vi "Analyze.vi"(8 "error in (no error)":errorcluster, 11 "HIJ Vision Display in":refnum<class "HIJ Vision Display.lvclass">) -> (0 "error out":errorcluster, 3 "HIJ Vision Display out":refnum<class "HIJ Vision Display.lvclass">)   [LabVIEW 2014, in "HIJ Vision Display.lvlib" / "HIJ Vision Display.lvclass"]
uses:
  HIJ Vision Display.lvclass
  <vilib>/vision/Image Controls.llb/IMAQ Image.ctl
  HIJ Vision Display.lvclass/HIJ Vision Display.ctl
  Analyze Actor/Analyze Actor Messages/Analyze Msg/Analyze Msg.lvclass/Analyze Msg.ctl
  <vilib>/ActorFramework/Message Enqueuer/Message Enqueuer.lvclass/Message Enqueuer.ctl
  <vilib>/ActorFramework/Message Enqueuer/Enqueue.vi
  <vilib>/ActorFramework/Message Priority Queue/Priority Enqueue.vi
  <vilib>/ActorFramework/Message Enqueuer/Message Enqueuer.lvclass
  Analyze Actor/Analyze Actor Messages/Analyze Msg/Analyze Msg.lvclass
panel:
  out "Image Out":T1
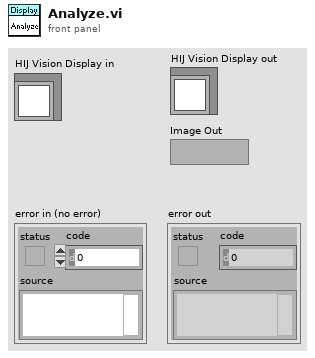
[diagram p1: front panel]
types:
  T1 = typedef "IMAQ Image.ctl" = refnum<image>
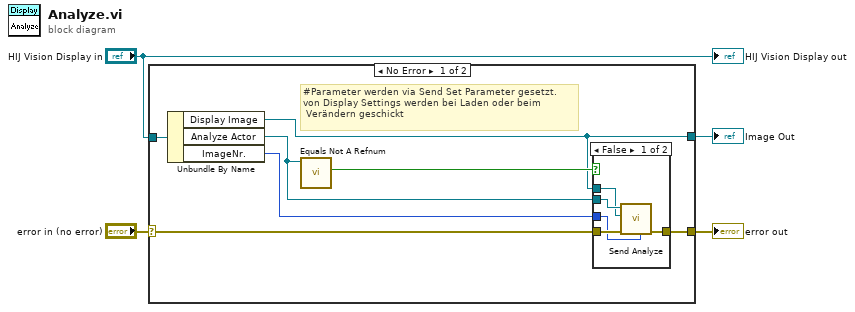
[diagram p0: block diagram]
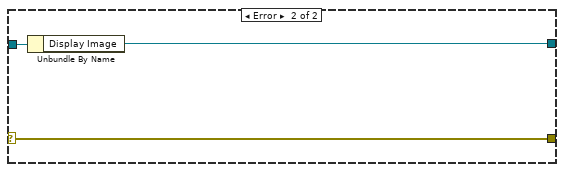
[diagram p3: hidden frame]
diagram:
  n1 = case shown="No Error" "error in (no error)" {
    selector: "error in (no error)" -> [w7 w20]
    tunnel: [w11 w20] -> w4
    tunnel: "HIJ Vision Display in" -> [w8 w19]
    tunnel: [w5 w18] -> w1
    frame No Error {
      # "#Parameter werden via Send Set Parameter gesetzt.\nvon Display Settings werden bei Laden oder beim\n Verändern geschickt"
      n2 = Unbundle By Name(w8) -> ("Display Image"=w5:T1, "Analyze Actor"=w10:refnum<class "Message Enqueuer.lvclass">, "ImageNr."=w9:i32)
      n3 = call <vilib>:"Equals Not A Refnum.vi"("Message Enqueuer"=w10) -> ("Not a refnum?"=w6:bool)  [unwired: 10 in]
      n4 = case shown="False" w6 {
        tunnel: w10 -> [w16 _]
        tunnel: w5 -> [w15 _]
        tunnel: w7 -> [w14 w17]
        tunnel: [w13 w17] -> w11
        tunnel: w9 -> [w12 _]
        frame False {
          n5 = call "Send Analyze.vi"("Image Nr."=w12, "error in (no error)"=w14, "Image"=w15, "Message Enqueuer"=w16) -> ("error out"=w13:errorcluster)  [unwired: 6 in, 1 out]
        }
        frame True {
        }
      }
    }
    frame Error {
      n6 = Unbundle By Name(w19) -> ("Display Image"=w18:T1)
    }
  }
  "error out" <- w4
  "Image Out" <- w1
  "HIJ Vision Display out" <- "HIJ Vision Display in"
